vi "Initialize.vi"(8 "error in (no error)":errorcluster, 9 "Reset (True)":bool=TRUE, 10 "ID Query (True)":bool=TRUE, 11 "VISA resource name":refnum<visa-resource-name>) -> (0 "error out":errorcluster, 3 "VISA resource name out":refnum<visa-resource-name>)   [LabVIEW 2017, in "Sefram DAS220.lvlib"]
doc: "Establishes communication with the instrument and optionally performs an instrument identification query and/or an instrument reset. It also places the instrument in a default state needed for other instrument driver operations. Therefore, call this VI before calling other instrument driver VIs for this instrument. Generally, you need to call the <b>Initialize</b> VI only once at the beginning of an application."
uses:
  <instrlib>/Sefram DAS220/Sefram DAS220.lvlib
panel:
  # "(c) 2017 Sefram Instruments.  ALL RIGHTS RESERVED."
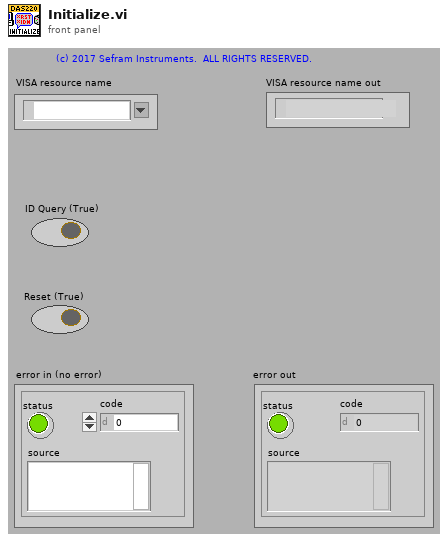
[diagram p1: front panel]
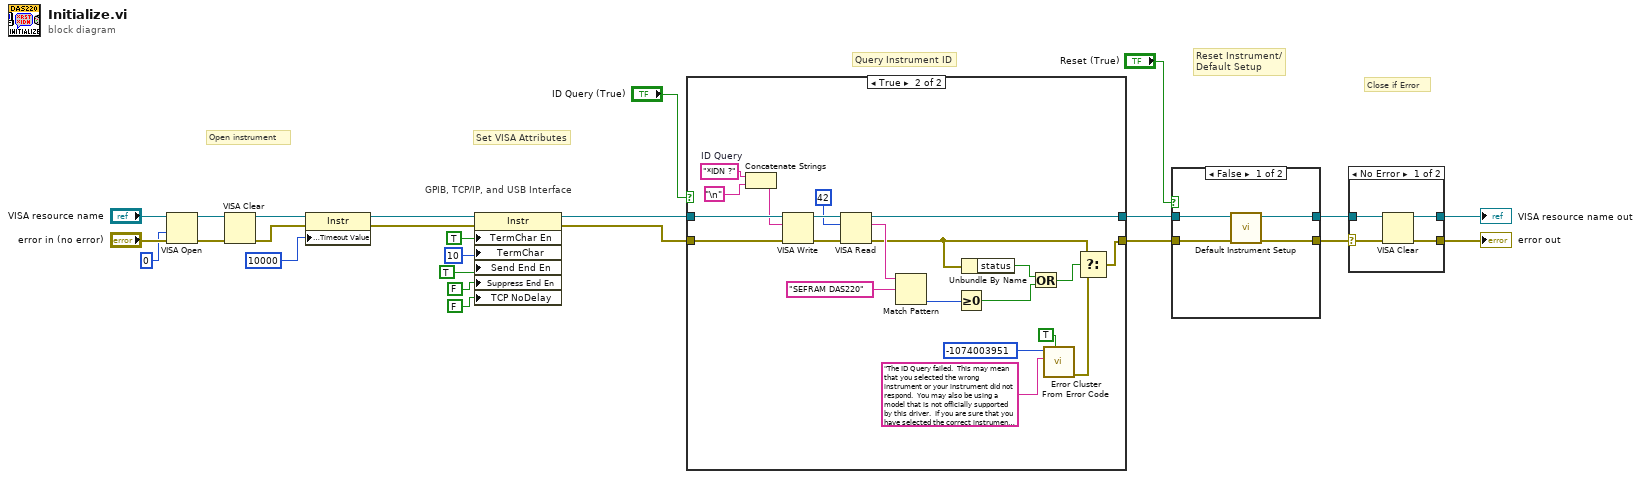
[diagram p0: block diagram]
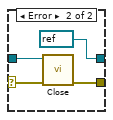
[diagram p2: hidden frame]
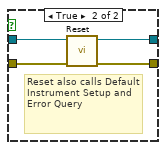
[diagram p3: hidden frame]
diagram:
  # "GPIB, TCP/IP, and USB Interface"
  # "Set VISA Attributes"
  # "Close if Error"
  # "Query Instrument ID"
  # "Reset Instrument/\nDefault Setup"
  # "Open instrument"
  n1 = VISA Open(access mode=u32 0, error in (no error)="error in (no error)", VISA resource name="VISA resource name") -> (VISA resource name=w4:refnum<visa-resource-name>, error out=w2:errorcluster)  [unwired: 2 in]
  n2 = VISA Clear(VISA resource name=w4, error in (no error)=w2) -> (VISA resource name out=w3:refnum<visa-resource-name>, error out=w1:errorcluster)
  n3 = property class="Instr"(reference=w3, error in=w1, "General Settings:Timeout Value"=u32 10000) -> (reference out=w13:refnum<visa-resource-name>, error out=w12:errorcluster)
  n4 = property class="Instr"(reference=w13, error in=w12, "TermChar En"=TRUE ("Message Based Settings:Termination Character Enable"), "TermChar"=u8 10 ("Message Based Settings:Termination Character"), "Send End En"=TRUE ("Message Based Settings:Send End Enable"), "Suppress End En"=FALSE ("Message Based Settings:Suppress End Enable"), "TCP NoDelay"=FALSE ("TCP/IP Settings:No Packet Delay")) -> (reference out=w11:refnum<visa-resource-name>, error out=w10:errorcluster)
  n5 = case shown="True" "ID Query (True)" {
    tunnel: [w26 w48] -> w24
    tunnel: [w27 w45] -> w25
    tunnel: w11 -> [w27 w46]
    tunnel: w10 -> [w26 w47]
    frame False {
    }
    frame True {
      w29 = "*IDN ?"  # ID Query
      n6 = Concatenate Strings(w29, "\n") -> (w30:string)
      n7 = VISA Write(VISA resource name=w46, write buffer=w30, error in (no error)=w47) -> (VISA resource name out=w43:refnum<visa-resource-name>, error out=w42:errorcluster)  [unwired: 1 out]
      n8 = VISA Read(VISA resource name=w43, byte count=u32 42, error in (no error)=w42) -> (VISA resource name out=w45:refnum<visa-resource-name>, read buffer=w44:string, error out=w34:errorcluster)  [unwired: 1 out]
      n9 = Match Pattern(string=w44, regular expression="SEFRAM DAS220") -> (offset past match=w35:i32)  [unwired: 1 in, 3 out]
      n10 = Greater Or Equal To 0?(x=w35) -> (x >= 0?=w32:bool)
      n11 = Unbundle By Name(w34) -> ("status"=w33:bool)
      n12 = Or(x=w33, y=w32) -> (x .or. y?=w31:bool)
      n13 = call <vilib>:"Error Cluster From Error Code.vi"("show call chain? (False)"=TRUE, "error message (\"\")"="The ID Query failed.  This may mean that you selected the wrong instrument or your instrument did not respond.  You may also be using a model that is not officially supported by this driver.  If you are sure that you have selected the correct instrument and it is responding, try disabling the ID Query." ("Source (VI Name)"), "error code (0)"=-1074003951 ("Code")) -> ("error out"=w39:errorcluster)  [unwired: 6 in]
      n14 = Select(t=w34, s=w31, f=w39) -> (s? t:f=w48:errorcluster)
    }
  }
  n15 = case shown="False" "Reset (True)" {
    tunnel: w24 -> [w51 w53]
    tunnel: [w49 w56] -> w14
    tunnel: w25 -> [w52 w54]
    tunnel: [w50 w55] -> w15
    frame False {
      n16 = call <instrlib>:"Default Instrument Setup.vi"("error in (no error)"=w51, "VISA resource name"=w52) -> ("error out"=w49:errorcluster, "VISA resource name out"=w50:refnum<visa-resource-name>)  [unwired: 8 in]
    }
    frame True {
      # "Reset also calls Default Instrument Setup and Error Query"
      n17 = call <instrlib>:"Reset.vi"("error in (no error)"=w53, "VISA resource name"=w54) -> ("error out"=w56:errorcluster, "VISA resource name out"=w55:refnum<visa-resource-name>)  [unwired: 8 in]
    }
  }
  n18 = case shown="No Error" w14 {
    selector: w14 -> [w59 w62]
    tunnel: w15 -> [w60 w63]
    tunnel: [w57 refnum<visa-resource-name> refnum ("VISA resource name out")] -> w17
    tunnel: [w58 w64] -> w16
    frame No Error {
      n19 = VISA Clear(VISA resource name=w60, error in (no error)=w59) -> (VISA resource name out=w57:refnum<visa-resource-name>, error out=w58:errorcluster)
    }
    frame Error {
      n20 = call <instrlib>:"Close.vi"("error in (no error)"=w62, "VISA resource name"=w63) -> ("error out"=w64:errorcluster)  [unwired: 9 in]
    }
  }
  "VISA resource name out" <- w17
  "error out" <- w16
